vi "Q.Return Function Data.vi"(8 "error in":errorcluster, 9 "Data2":variant, 11 "Ret Data":variant) -> (0 "error out":errorcluster)   [LabVIEW 2024, in "EQMF.lvlib" / "Queue Utils.lvlib"]
uses:
  Queue Utils.lvlib
  Q.Msg Return Info.ctl
  Q.Element.ctl
  Q.Msg Return Data Container.ctl
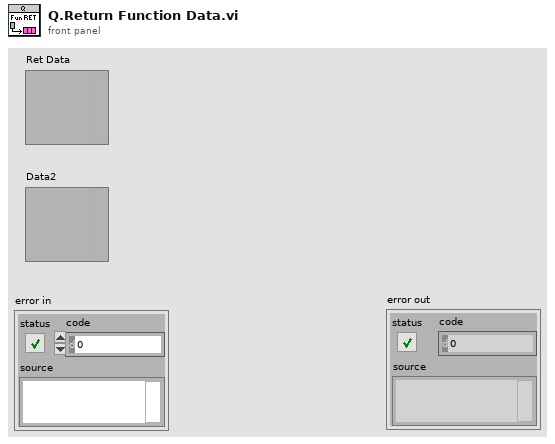
[diagram p1: front panel]
types:
  T1 = typedef "EQMF.lvlib/Queue Utils.lvlib/Q.Msg Return Info.ctl" = cluster{"Ret Q":refnum<queue>, "Ret Msg":T2, "SeqNum":i32}
  T2 = typedef "EQMF.lvlib/Queue Utils.lvlib/Q.Element.ctl" = cluster{"Cmd":string, "Sub":string, "Data1":variant, "Data2":variant}
  T3 = typedef "EQMF.lvlib/Queue Utils.lvlib/Q.Msg Return Data Container.ctl" = cluster{"SeqNum":i32, "Data":variant, "Error":errorcluster}
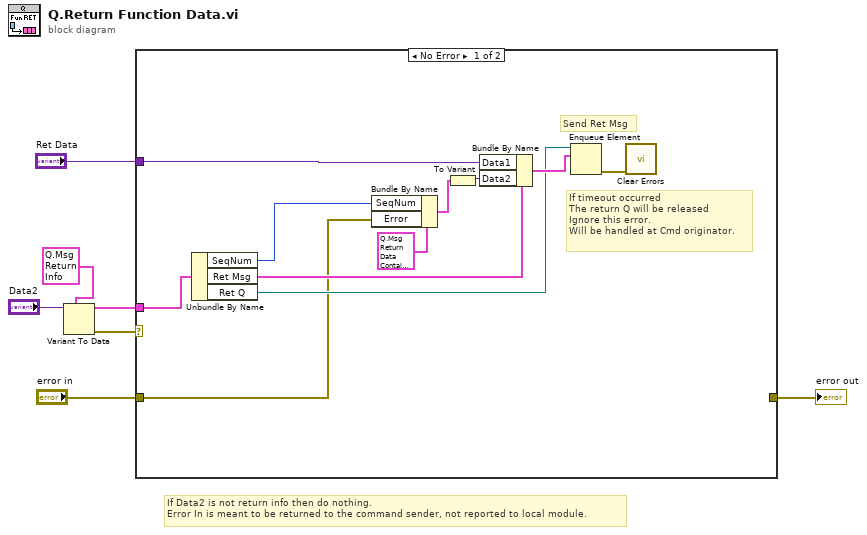
[diagram p0: block diagram]
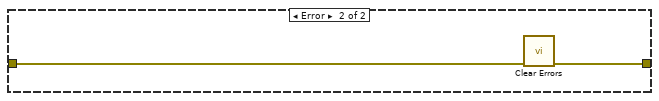
[diagram p2: hidden frame]
diagram:
  # "If Data2 is not return info then do nothing.\nError In is meant to be returned to the command sender, not reported to local module."
  n1 = Variant To Data(type=T1 {"Ret Q"=refnum, "Ret Msg"={"Cmd"="", "Sub"="", "Data1"=variant, "Data2"=variant}, "SeqNum"=0} ("Cmd Ret Req Data"), Variant="Data2") -> (data=w6:T1, error out=w1:errorcluster)  [unwired: 1 in]
  n2 = case shown="No Error" w1 {
    tunnel: w6 -> [w18 _]
    tunnel: "Ret Data" -> [w10 _]
    tunnel: "error in" -> [w9 w19]
    tunnel: [_ w20] -> w2
    frame No Error {
      # "If timeout occurred\nThe return Q will be released\nIgnore this error.\nWill be handled at Cmd originator."
      # "Send Ret Msg"
      n3 = Unbundle By Name(w18) -> ("SeqNum"=w13:i32, "Ret Msg"=w17:T2, "Ret Q"=w15:refnum<queue>)
      n4 = Bundle By Name(cluster=T3 {"SeqNum"=0, "Data"=variant, "Error"={"status"=FALSE, "code"=0, "source"=""}} ("Ret"), "SeqNum"=w13, "Error"=w9) -> (w11:T3)
      n5 = To Variant(anything=w11) -> (Variant=w12:variant)
      n6 = Bundle By Name(cluster=w17, "Data1"=w10, "Data2"=w12) -> (w16:T2)
      n7 = Enqueue Element(queue=w15, element=w16) -> (error out=w8:errorcluster)  [unwired: 2 in, 2 out]
      n8 = call <vilib>:"Clear Errors.vi"("error in (no error)"=w8) -> ()  [unwired: 5 in, 2 out]
    }
    frame Error {
      n9 = call <vilib>:"Clear Errors.vi"("error in (no error)"=w19) -> ("error out"=w20:errorcluster)  [unwired: 5 in, 1 out]
    }
  }
  "error out" <- w2
